vi "Config Menu.vi"(5 "Stats":string[][](table) caption="Result Set (from first statement with results)", 7 "Data Out":string[][](table) caption="Result Set (from first statement with results)", 8 "error in (no error)":errorcluster, 11 "Enum":enum16{"Initial Menu", "Final Menu"}(ring)) -> (0 "error out":errorcluster, 1 "Play/stop":bool, 3 "output cluster":refnum<class "Application.lvclass">)   [LabVIEW 2021, in "Application.lvclass"]
uses:
  Application/Application.lvclass
  <vilib>/Utility/miscctls.llb/LVRowAndColumnTypeDef.ctl
  Application/Application.lvclass/Application.ctl
  Application/Globales Snake.vi
  <vilib>/sound2/lvsound2.llb/Sound Output Set Volume (Single).vi
panel:
  out "GAME STATS":bool
  in  "GAME STATS":i32(listbox)
  out "LEADERBOARD":bool
  in  "Player Name":string="user"
  out "Instructions":bool
  out "INSTRUCTIONS":bool
  in  "Stop":bool
  in  "Start Game":bool
  in  "LEADERBOARD":i32(listbox)
  in  "Number of Bombs":i32=1
  in  "Play with Bombs":bool
  in  "Music:":u32(ring) items=["Music 1", "Music 2", "Music 3", "Music 4"]
  in  "Game Difficulty:":u32(ring)=150 items=["Easy"=750, "Hard"=500, "Extreme"=300, "Carlo Music"=150]
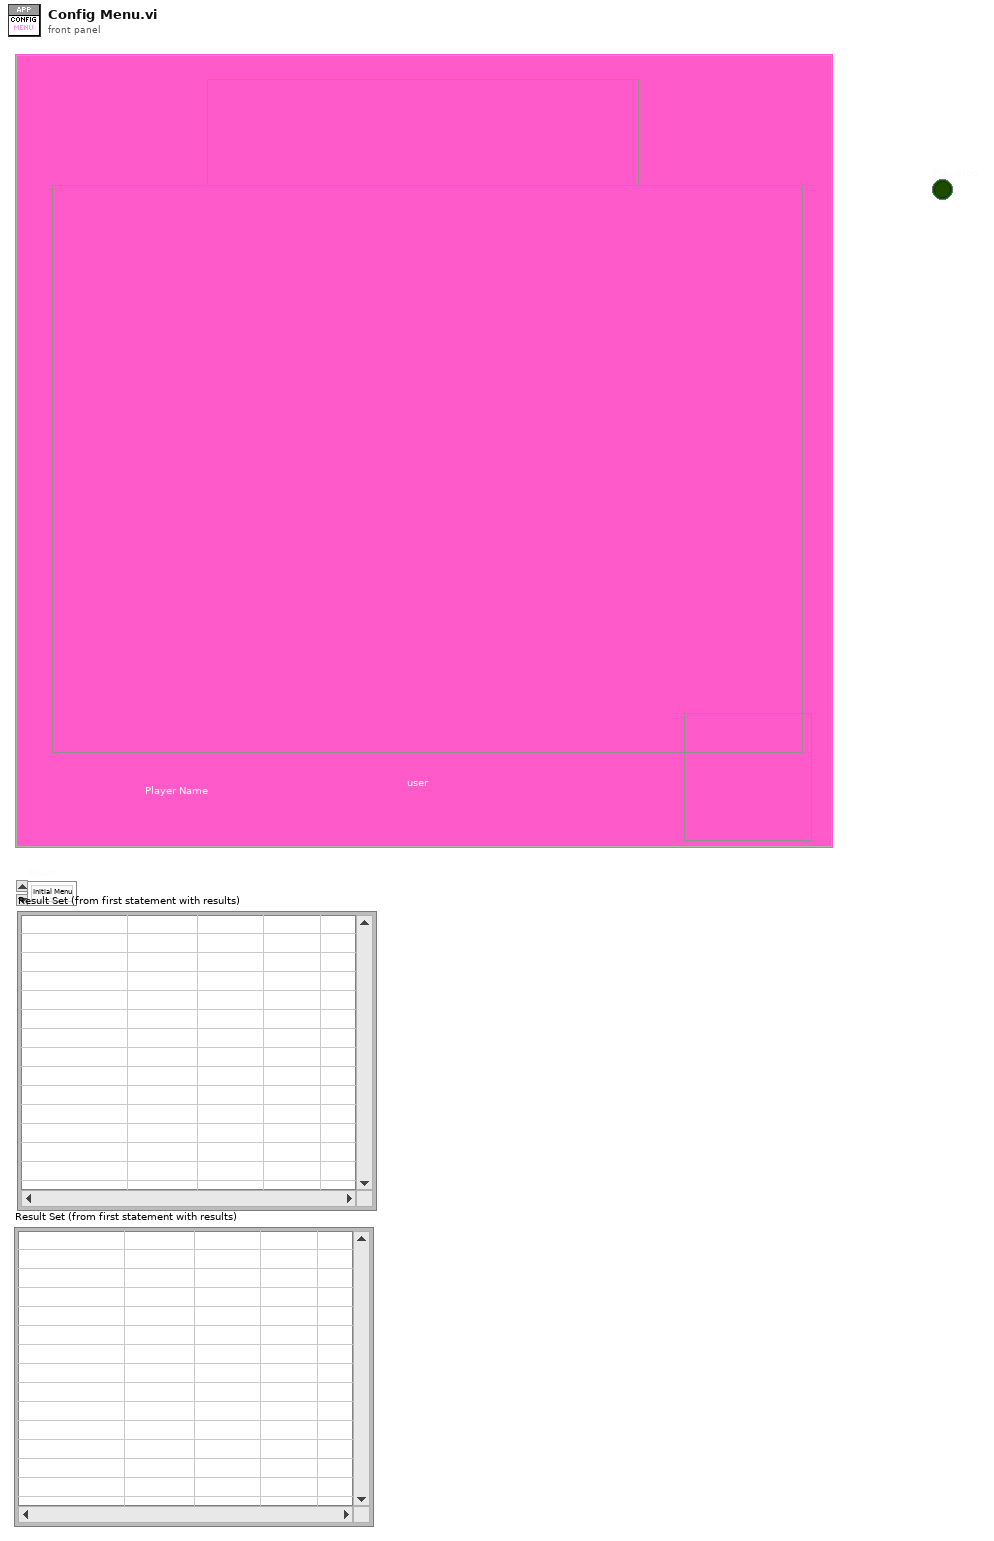
[diagram p1: front panel]
types:
  T1 = typedef "LVRowAndColumnTypeDef.ctl" = cluster{"Row":i32, "Column":i32}
  T2 = cluster{"Music:":u32, "Game Difficulty:":u32, "Number of Bombs":i32}
  T3 = enum32{"Invalid", "Standard", "Closed", "Hidden", "Minimized", "Maximized"}
  T4 = typedef "Sound Output Task ID.ctl" = u32
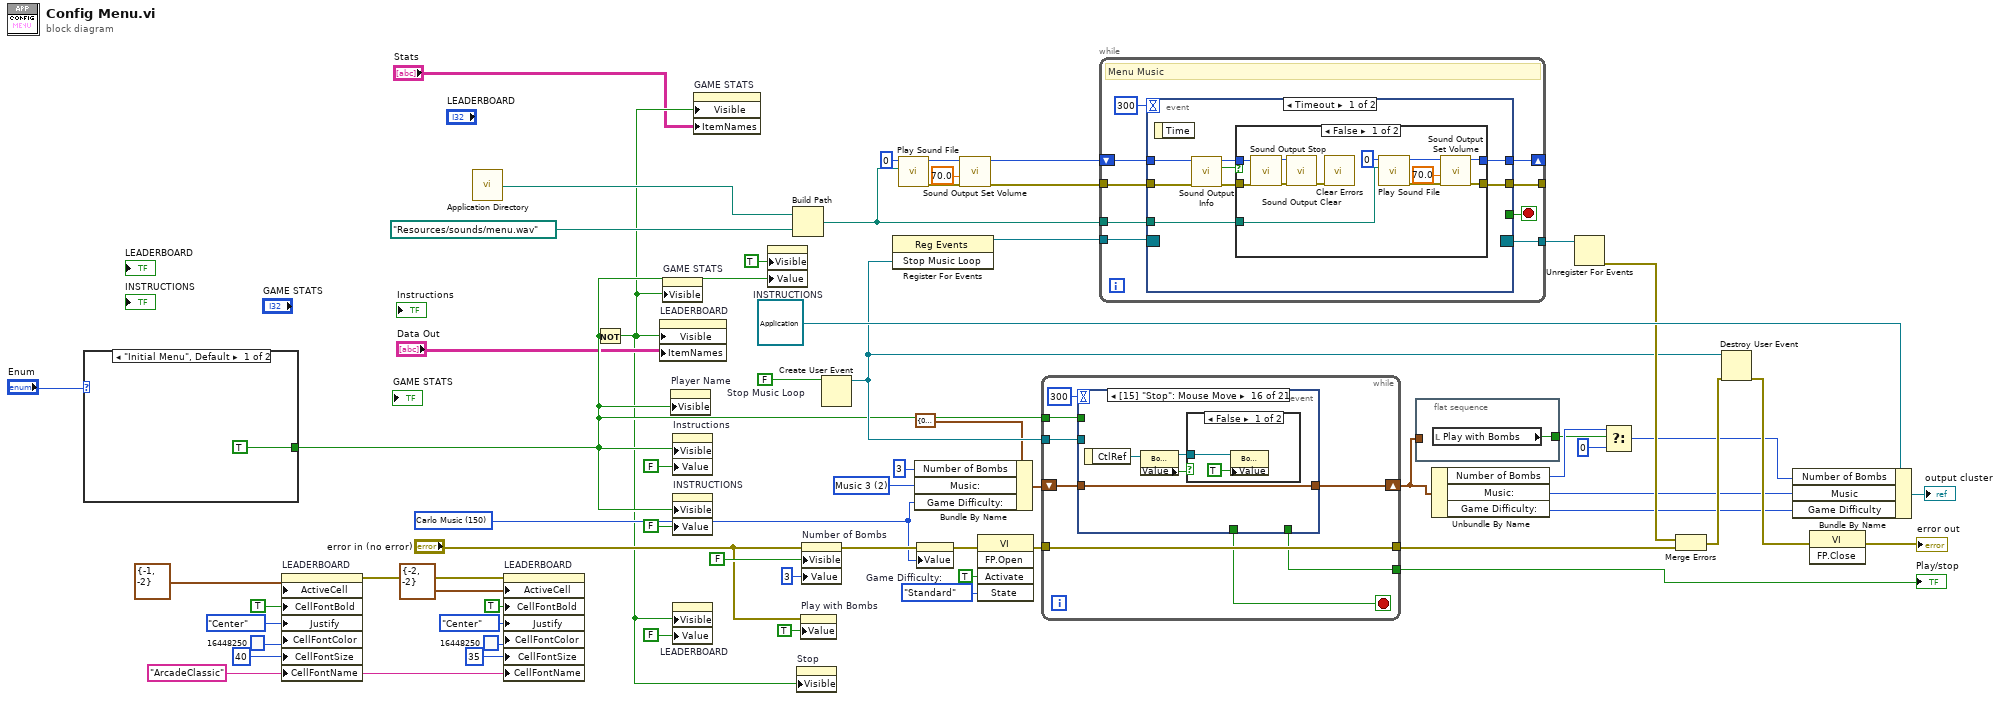
[diagram p0: block diagram]
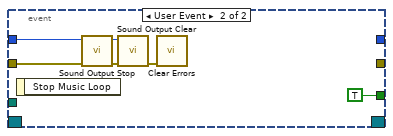
[diagram p4: hidden frame]
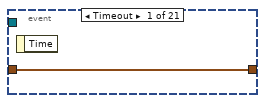
[diagram p5: hidden frame]
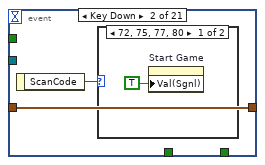
[diagram p6: hidden frame]
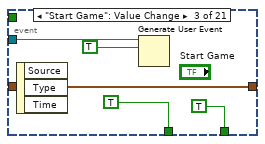
[diagram p8: hidden frame]
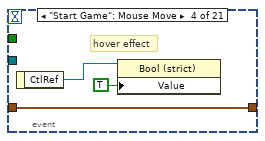
[diagram p9: hidden frame]
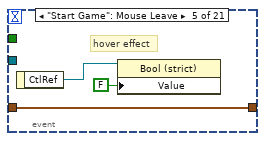
[diagram p10: hidden frame]
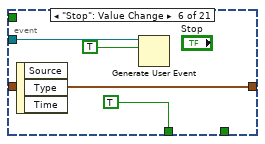
[diagram p11: hidden frame]
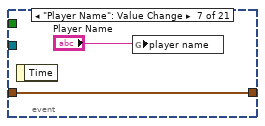
[diagram p12: hidden frame]
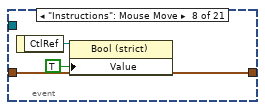
[diagram p13: hidden frame]
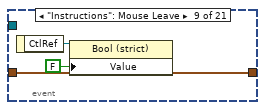
[diagram p14: hidden frame]
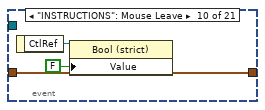
[diagram p15: hidden frame]
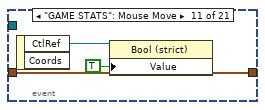
[diagram p16: hidden frame]
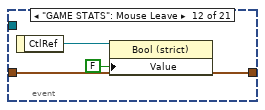
[diagram p17: hidden frame]
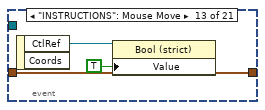
[diagram p18: hidden frame]
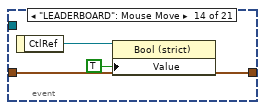
[diagram p19: hidden frame]
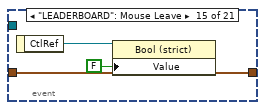
[diagram p20: hidden frame]
diagram:
  w3 = "ArcadeClassic" ("Active Cell:Cell Font:Name")
  w30 = u32 150 items=["Easy"=750, "Hard"=500, "Extreme"=300, "Carlo Music"=150] ("Game Difficulty:")
  w57 = FALSE  # Stop Music Loop
  w31 = u32 2 items=["Music 1", "Music 2", "Music 3", "Music 4"] ("Music:")
  n1 = case shown="\"Initial Menu\", Default" "Enum" {
    tunnel: [TRUE ("Visible") _] -> w5
    frame "Initial Menu", Default {
    }
    frame "Final Menu" {
    }
  }
  n2 = property on="LEADERBOARD" class="MCListbox (strict)"("ActiveCell"=T1 {"Row"=-1, "Column"=-2} ("Active Cell:Active Cell"), "CellFontBold"=TRUE ("Active Cell:Cell Font:Bold"), "Justify"=enum16{"Left", "Center", "Right"}."Center" ("Active Cell:Cell Justification"), "CellFontColor"=u32 16448250 ("Active Cell:Cell Font:Color"), "CellFontSize"=u32 40 ("Active Cell:Cell Font:Size"), "CellFontName"=w3) -> (error out=w6:errorcluster)  [unwired: 2 in, 1 out]
  n3 = call <vilib>:"Application Directory.vi"() -> ("Application Directory"=w50:path)
  n4 = property on="LEADERBOARD" class="MCListbox (strict)"(error in=w6, "ActiveCell"=T1 {"Row"=-2, "Column"=-2} ("Active Cell:Active Cell"), "CellFontBold"=TRUE ("Active Cell:Cell Font:Bold"), "Justify"=enum16{"Left", "Center", "Right"}."Center" ("Active Cell:Cell Justification"), "CellFontColor"=u32 16448250 ("Active Cell:Cell Font:Color"), "CellFontSize"=u32 35 ("Active Cell:Cell Font:Size"), "CellFontName"=w3) -> ()  [unwired: 1 in, 2 out]
  n5 = Not(x=w5) -> (.not. x?=w2:bool)
  n6 = property on="LEADERBOARD" class="MCListbox (strict)"("Visible"=w2, "ItemNames"="Data Out") -> ()  [unwired: 2 in, 2 out]
  n7 = property on="GAME STATS" class="Bool (strict)"("Visible"=w2) -> ()  [unwired: 2 in, 2 out]
  n8 = property on="Player Name" class="Str"("Visible"=w5) -> ()  [unwired: 2 in, 2 out]
  n9 = property on="Instructions" class="Bool (strict)"("Visible"=w5, "Value"=FALSE ("Instructions")) -> ()  [unwired: 2 in, 2 out]
  n10 = property on="INSTRUCTIONS" class="Bool (strict)"("Visible"=w5, "Value"=FALSE ("Instructions")) -> ()  [unwired: 2 in, 2 out]
  n11 = property on="LEADERBOARD" class="Bool (strict)"("Visible"=w2, "Value"=FALSE ("Instructions")) -> ()  [unwired: 2 in, 2 out]
  n12 = property on="GAME STATS" class="MCListbox (strict)"("Visible"=w2, "ItemNames"="Stats") -> ()  [unwired: 2 in, 2 out]
  n13 = property on="INSTRUCTIONS" class="Bool (strict)"("Visible"=TRUE, "Value"=w5) -> ()  [unwired: 2 in, 2 out]
  n14 = Build Path(base path=w50, name or relative path=path "Resources/sounds/menu.wav") -> (appended path=w48:path)
  n15 = property on="Stop" class="Bool (strict)"("Visible"=w2) -> ()  [unwired: 2 in, 2 out]
  n16 = property on="Play with Bombs" class="Bool (strict)"(error in="error in (no error)", "Value"=TRUE ("Play with Bombs")) -> ()  [unwired: 1 in, 2 out]
  n17 = property on="Number of Bombs" class="DigNum (strict)"(error in="error in (no error)", "Visible"=FALSE, "Value"=3 ("Number of Bombs")) -> (error out=w39:errorcluster)  [unwired: 1 in, 1 out]
  n18 = Create User Event(user event datatype=w57) -> (user event=w44:refnum<user-event>)  [unwired: 1 in, 1 out]
  n19 = register-events(w44) -> (reference out=w47:refnum<event-registration>)  [unwired: 2 in, 1 out]
  n20 = call <vilib>:"Play Sound File.vi"("path"=w48, "device ID"=u32 0) -> ("error out"=w55:errorcluster, "task ID"=w54:T4)  [unwired: 8 in]
  n21 = Bundle By Name(cluster=T2 {"Music:"=0, "Game Difficulty:"=150, "Number of Bombs"=1}, "Number of Bombs"=3, "Music:"=w31, "Game Difficulty:"=w30) -> (w29:T2)
  n22 = property on="Game Difficulty:" class="Ring (strict)"(error in=w39, "Value"=w30) -> (error out=w41:errorcluster)  [unwired: 1 in, 1 out]
  n23 = call-poly <vilib>:"Sound Output Set Volume.vi"("error in (no error)"=w55, "volume"=70.0, "task ID"=w54) -> ("error out"=w52:errorcluster, "task ID out"=w51:T4)  [unwired: 7 in]
  n24 = invoke class="VI" method="FP.Open"(error in=w41, "Activate"=TRUE ("Activate?"), "State"=T3."Standard") -> (error out=w40:errorcluster)  [unwired: 2 in, 4 out]
  n25 = while {
    tunnel: w40 -> [w72]
    tunnel: [w72] -> w61
    shift-right: [w69] -> w25
    shift-left: w29 -> [w70]
    tunnel: w44 -> [w68]
    tunnel: [w67] -> w21
    tunnel: w5 -> [w65]
    stop <- w71 stop-if-true
    n26 = event shown="[15] \"Stop\": Mouse Move" {
      selector: _ -> [_ _ _ _ _ _ _ _ _ _ _ _ _ _ _ _ _ _ _ _ _]
      dyn-events: _ -> [_ _ _ _ _ _ _ _ _ _ _ _ _ _ _ _ _ _ _ _ _]
      timeout: 300 -> [_ _ _ _ _ _ _ _ _ _ _ _ _ _ _ _ _ _ _ _ _]
      tunnel: [_ _ TRUE _ _ TRUE _ _ _ _ _ _ _ _ _ _ _ _ _ _ _] -> w71
      tunnel: w70 -> [w73 w75 w80 w84 w87 w90 w93 w96 w99 w102 w105 w108 w111 w114 w117 w121 w127 w132 w134 w137 w140]
      tunnel: [w73 w75 w80 w84 w87 w90 w93 w96 w99 w102 w105 w108 w111 w114 w117 w121 w127 w131 w135 w137 w139] -> w69
      tunnel: w68 -> [_ _ w79 _ _ w89 _ _ _ _ _ _ _ _ _ _ _ _ _ _ _]
      tunnel: [_ _ TRUE _ _ _ _ _ _ _ _ _ _ _ _ _ _ _ _ _ _] -> w67
      tunnel: w65 -> [_ _ _ _ _ _ _ _ _ _ _ _ _ _ _ _ _ _ _ _ _]
      event Timeout {
        n27 = event-data() -> ()  [unwired: 1 in, 1 out]
      }
      event Key Down {
        n28 = event-data() -> ("ScanCode"=w74:i16)  [unwired: 1 in]
        n29 = case shown="72, 75, 77, 80" w74 {
          frame 72, 75, 77, 80 {
            n30 = property on="Start Game" class="Bool (strict)"("Val(Sgnl)"=TRUE ("Value (Signaling)")) -> ()  [unwired: 2 in, 2 out]
          }
          frame Default {
          }
        }
      }
      event "Start Game": Value Change {
        n31 = event-data() -> ()  [unwired: 1 in, 3 out]
        n32 = Generate User Event(user event=w79, event data cluster=TRUE ("event data")) -> ()  [unwired: 2 in, 2 out]
      }
      event "Start Game": Mouse Move {
        # "hover effect"
        n33 = event-data() -> ("CtlRef"=w83:refnum<vi>)  [unwired: 1 in]
        n34 = property class="Bool (strict)"(reference=w83, "Value"=TRUE) -> ()  [unwired: 1 in, 2 out]
      }
      event "Start Game": Mouse Leave {
        # "hover effect"
        n35 = event-data() -> ("CtlRef"=w86:refnum<vi>)  [unwired: 1 in]
        n36 = property class="Bool (strict)"(reference=w86, "Value"=FALSE) -> ()  [unwired: 1 in, 2 out]
      }
      event "Stop": Value Change {
        n37 = event-data() -> ()  [unwired: 1 in, 3 out]
        n38 = Generate User Event(user event=w89, event data cluster=TRUE ("event data")) -> ()  [unwired: 2 in, 2 out]
      }
      event "Player Name": Value Change {
        n39 = event-data() -> ()  [unwired: 1 in, 1 out]
        n40 = global write "Globales Snake.vi" "player name"("Player Name") -> ()
      }
      event "Instructions": Mouse Move {
        n41 = event-data() -> ("CtlRef"=w95:refnum<vi>)  [unwired: 1 in]
        n42 = property class="Bool (strict)"(reference=w95, "Value"=TRUE) -> ()  [unwired: 1 in, 2 out]
      }
      event "Instructions": Mouse Leave {
        n43 = event-data() -> ("CtlRef"=w98:refnum<vi>)  [unwired: 1 in]
        n44 = property class="Bool (strict)"(reference=w98, "Value"=FALSE) -> ()  [unwired: 1 in, 2 out]
      }
      event "INSTRUCTIONS": Mouse Leave {
        n45 = event-data() -> ("CtlRef"=w101:refnum<vi>)  [unwired: 1 in]
        n46 = property class="Bool (strict)"(reference=w101, "Value"=FALSE) -> ()  [unwired: 1 in, 2 out]
      }
      event "GAME STATS": Mouse Move {
        n47 = event-data() -> ("CtlRef"=w104:refnum<vi>)  [unwired: 1 in, 1 out]
        n48 = property class="Bool (strict)"(reference=w104, "Value"=TRUE) -> ()  [unwired: 1 in, 2 out]
      }
      event "GAME STATS": Mouse Leave {
        n49 = event-data() -> ("CtlRef"=w107:refnum<vi>)  [unwired: 1 in]
        n50 = property class="Bool (strict)"(reference=w107, "Value"=FALSE) -> ()  [unwired: 1 in, 2 out]
      }
      event "INSTRUCTIONS": Mouse Move {
        n51 = event-data() -> ("CtlRef"=w110:refnum<vi>)  [unwired: 1 in, 1 out]
        n52 = property class="Bool (strict)"(reference=w110, "Value"=TRUE) -> ()  [unwired: 1 in, 2 out]
      }
      event "LEADERBOARD": Mouse Move {
        n53 = event-data() -> ("CtlRef"=w113:refnum<vi>)  [unwired: 1 in]
        n54 = property class="Bool (strict)"(reference=w113, "Value"=TRUE) -> ()  [unwired: 1 in, 2 out]
      }
      event "LEADERBOARD": Mouse Leave {
        n55 = event-data() -> ("CtlRef"=w116:refnum<vi>)  [unwired: 1 in]
        n56 = property class="Bool (strict)"(reference=w116, "Value"=FALSE) -> ()  [unwired: 1 in, 2 out]
      }
      event "Stop": Mouse Move {
        n57 = event-data() -> ("CtlRef"=w120:refnum<vi>)  [unwired: 1 in]
        n58 = property class="Bool (strict)"(reference=w120) -> (reference out=w118:refnum<vi>, "Value"=w119:bool)  [unwired: 1 in, 1 out]
        n59 = case shown="False" w119 {
          tunnel: w118 -> [w123 _]
          frame False {
            n60 = property class="Bool (strict)"(reference=w123, "Value"=TRUE) -> ()  [unwired: 1 in, 2 out]
          }
          frame True {
          }
        }
      }
      event "Stop": Mouse Leave {
        n61 = event-data() -> ("CtlRef"=w126:refnum<vi>)  [unwired: 1 in]
        n62 = property class="Bool (strict)"(reference=w126) -> (reference out=w124:refnum<vi>, "Value"=w125:bool)  [unwired: 1 in, 1 out]
        n63 = case shown="True" w125 {
          tunnel: w124 -> [_ w129]
          frame False {
          }
          frame True {
            n64 = property class="Bool (strict)"(reference=w129, "Value"=FALSE) -> ()  [unwired: 1 in, 2 out]
          }
        }
      }
      event "Game Difficulty:": Value Change {
        n65 = event-data() -> ("NewVal"=w130:u32)  [unwired: 1 in]
        n66 = Bundle By Name(cluster=w132, "Game Difficulty:"=w130) -> (w131:T2)
      }
      event "Music:": Value Change {
        n67 = event-data() -> ()  [unwired: 1 in, 1 out]
        n68 = Bundle By Name(cluster=w134, "Music:"="Music:") -> (w135:T2)
      }
      event "Play with Bombs": Value Change {
        n69 = event-data() -> ("NewVal"=w136:bool)  [unwired: 1 in]
        n70 = property on="Number of Bombs" class="DigNum (strict)"("Visible"=w136) -> ()  [unwired: 2 in, 2 out]
      }
      event "Number of Bombs": Value Change {
        n71 = event-data() -> ()  [unwired: 1 in, 1 out]
        n72 = Bundle By Name(cluster=w140, "Number of Bombs"="Number of Bombs") -> (w139:T2)
      }
    }
  }
  "Play/stop" <- w21
  n73 = while {
    tunnel: w52 -> [w148]
    shift-right: [w146] -> _
    shift-left: w51 -> [w147]
    tunnel: [w145] -> _
    tunnel: w48 -> [w144]
    tunnel: w47 -> [w143]
    tunnel: [w142] -> w46
    stop <- w141 stop-if-true
    # "Menu Music"
    n74 = event shown="[0] Timeout" {
      selector: w143 -> [_ _]
      dyn-events: [_ _] -> w142
      timeout: 300 -> [_ _]
      tunnel: w148 -> [w156 w173]
      tunnel: w147 -> [w157 w174]
      tunnel: [w152 _] -> w146
      tunnel: [w151 _] -> w145
      tunnel: w144 -> [w150 _]
      tunnel: [_ TRUE] -> w141
      event Timeout {
        n75 = event-data() -> ()  [unwired: 1 in, 1 out]
        n76 = call <vilib>:"Sound Output Info.vi"("error in (no error)"=w156, "task ID"=w157) -> ("error out"=w155:errorcluster, "is playing?"=w154:bool, "task ID out"=w153:T4)  [unwired: 6 in, 1 out]
        n77 = case shown="False" w154 {
          tunnel: w155 -> [w167 w170]
          tunnel: w153 -> [w168 w171]
          tunnel: [w160 w171] -> w152
          tunnel: [w159 w170] -> w151
          tunnel: w150 -> [w158 _]
          frame False {
            n78 = call <vilib>:"Sound Output Stop.vi"("error in (no error)"=w167, "task ID"=w168) -> ("error out"=w165:errorcluster, "task ID out"=w169:T4)  [unwired: 8 in]
            n79 = call <vilib>:"Sound Output Clear.vi"("error in (no error)"=w165, "task ID"=w169) -> ("error out"=w166:errorcluster)  [unwired: 9 in]
            n80 = call <vilib>:"Clear Errors.vi"("error in (no error)"=w166) -> ()  [unwired: 5 in, 2 out]
            n81 = call <vilib>:"Play Sound File.vi"("path"=w158, "device ID"=u32 0) -> ("error out"=w162:errorcluster, "task ID"=w163:T4)  [unwired: 8 in]
            n82 = call-poly <vilib>:"Sound Output Set Volume.vi"("error in (no error)"=w162, "volume"=70.0, "task ID"=w163) -> ("error out"=w159:errorcluster, "task ID out"=w160:T4)  [unwired: 7 in]
          }
          frame True {
          }
        }
      }
      event User Event {
        n83 = event-data() -> ()  [unwired: 1 in, 1 out]
        n84 = call <vilib>:"Sound Output Stop.vi"("error in (no error)"=w173, "task ID"=w174) -> ("error out"=w175:errorcluster, "task ID out"=w177:T4)  [unwired: 8 in]
        n85 = call <vilib>:"Sound Output Clear.vi"("error in (no error)"=w175, "task ID"=w177) -> ("error out"=w176:errorcluster)  [unwired: 9 in]
        n86 = call <vilib>:"Clear Errors.vi"("error in (no error)"=w176) -> ()  [unwired: 5 in, 2 out]
      }
    }
  }
  n87 = flat-sequence {
    tunnel: w25 -> [_]
    tunnel: [w178] -> w24
    frame #0 {
      n88 = local read "Play with Bombs"() -> (w178:bool)
    }
  }
  n89 = Unbundle By Name(w25) -> ("Number of Bombs"=w26:i32, "Music:"=w28:u32, "Game Difficulty:"=w27:u32)
  n90 = Unregister For Events(event registration refnum=w46) -> (error out=w45:errorcluster)  [unwired: 1 in]
  n91 = Select(t=w26, s=w24, f=0) -> (s? t:f=w36:i32)
  n92 = Merge Errors(w45, w61) -> (w43:errorcluster)
  n93 = Destroy User Event(user event=w44, error in=w43) -> (error out=w42:errorcluster)
  n94 = Bundle By Name(cluster=refnum<class "Application.lvclass"> refnum ("Application.lvclass"), "Number of Bombs"=w36, "Music"=w28, "Game Difficulty"=w27) -> (→"output cluster":refnum<class "Application.lvclass">)
  n95 = invoke class="VI" method="FP.Close"(error in=w42) -> (error out=→"error out":errorcluster)  [unwired: 2 in, 2 out]
